vi "Configure Auto Port Extension Frequency.vi"(0 "VISA resource name":refnum<visa-resource-name>, 1 "Enable Loss Compensation (F: Disable)":bool, 2 "Enable DC Offset (F: Disable)":bool, 5 "Channel (1)":i32=1, 7 "Frequency Configuration (0: Current Sweep Range)":i32(ring) items=["Current Sweep Range", "Active Marker", "Arbitrary"], 11 "error in (no error)":errorcluster, 12 "Start Frequency (5)":dbl=5.0, 13 "Stop Frequency (3E+9 Hz)":dbl=3000000000.0) -> (4 "VISA resource name out":refnum<visa-resource-name>, 15 "error out":errorcluster)   [LabVIEW 2022 SP3, in "Agilent ENA Series.lvlib"]
doc: "Configures the auto port extension frequency settings.\n\n<B>Note:</B> This VI is only valid for E5061B, E5070B and E5071B."
uses:
  <instrlib>/Agilent ENA Series/Agilent ENA Series.lvlib
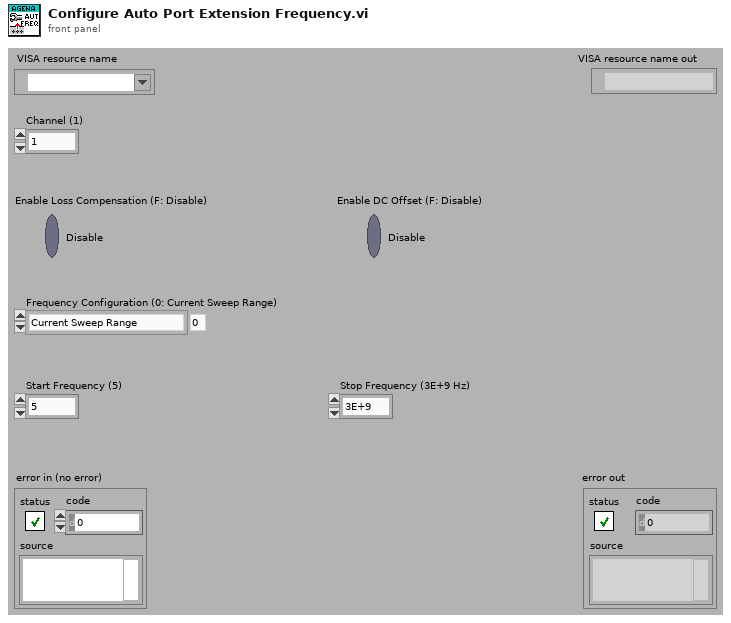
[diagram p1: front panel]
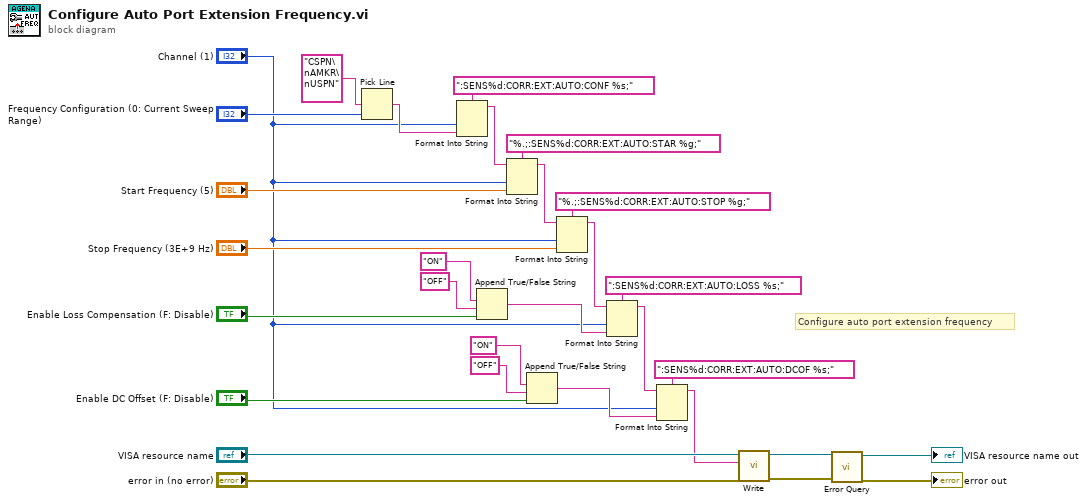
[diagram p0: block diagram]
diagram:
  # "Configure auto port extension frequency"
  n1 = Pick Line(multi-line string="CSPN\nAMKR\nUSPN", line index="Frequency Configuration (0: Current Sweep Range)") -> (output string=w27:string)  [unwired: 1 out]
  n2 = Format Into String(format string=":SENS%d:CORR:EXT:AUTO:CONF %s;", "Channel (1)", w27) -> (resulting string=w26:string)  [unwired: 2 in, 1 out]
  n3 = Append True/False String(1:"Enable Loss Compensation (F: Disable)", 2:"OFF", 3:"ON") -> (0:w15:string)  [unwired: 1 out]
  n4 = Format Into String(format string="%.;:SENS%d:CORR:EXT:AUTO:STAR %g;", initial string=w26, "Channel (1)", "Start Frequency (5)") -> (resulting string=w23:string)  [unwired: 1 in, 1 out]
  n5 = Append True/False String(1:"Enable DC Offset (F: Disable)", 2:"OFF", 3:"ON") -> (0:w9:string)  [unwired: 1 out]
  n6 = Format Into String(format string="%.;:SENS%d:CORR:EXT:AUTO:STOP %g;", initial string=w23, "Channel (1)", "Stop Frequency (3E+9 Hz)") -> (resulting string=w17:string)  [unwired: 1 in, 1 out]
  n7 = Format Into String(format string=":SENS%d:CORR:EXT:AUTO:LOSS %s;", initial string=w17, "Channel (1)", w15) -> (resulting string=w11:string)  [unwired: 1 in, 1 out]
  n8 = Format Into String(format string=":SENS%d:CORR:EXT:AUTO:DCOF %s;", initial string=w11, "Channel (1)", w9) -> (resulting string=w3:string)  [unwired: 1 in, 1 out]
  n9 = call <instrlib>:"Write.vi"("error in (no error)"="error in (no error)", "String ()"=w3, "VISA resource name"="VISA resource name") -> ("error out"=w1:errorcluster, "VISA resource name out"=w2:refnum<visa-resource-name>)  [unwired: 6 in, 1 out]
  n10 = call <instrlib>:"Error Query.vi"("error in (no error)"=w1, "VISA resource name"=w2) -> ("error out"=→"error out":errorcluster, "VISA resource name out"=→"VISA resource name out":refnum<visa-resource-name>)  [unwired: 8 out]
